vi "PM9_TCP_OPEN-SESSION.vi"(0 "VISA":refnum<visa-resource-name>="TCPIP0::169.254.70.190::502::SOCKET", 11 "error in (no error)":errorcluster) -> (6 "connection ID out":refnum<k5>, 15 "error out":errorcluster)   [LabVIEW 2018]
panel:
  in  "timeout ms ()":i32=5000
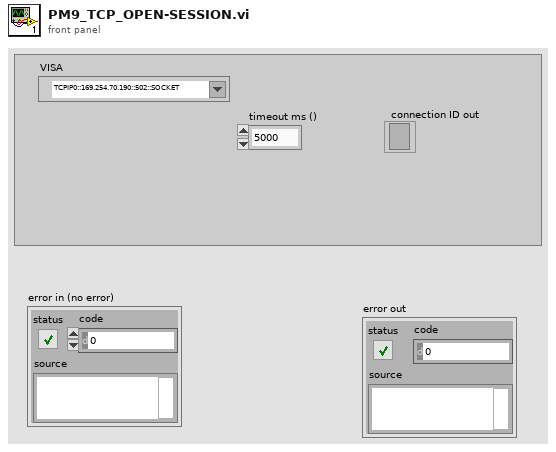
[diagram p1: front panel]
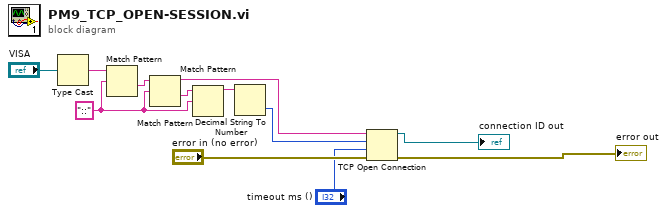
[diagram p0: block diagram]
diagram:
  w7 = "::" ("search string/char (-)")
  n1 = Type Cast(x="VISA") -> (*(type *) &x=w11:string)  [unwired: 1 in]
  n2 = Match Pattern(string=w11, regular expression=w7) -> (after substring=w10:string)  [unwired: 1 in, 3 out]
  n3 = Match Pattern(string=w10, regular expression=w7) -> (before substring=w9:string, after substring=w8:string)  [unwired: 1 in, 2 out]
  n4 = Match Pattern(string=w8, regular expression=w7) -> (before substring=w6:string)  [unwired: 1 in, 3 out]
  n5 = Decimal String To Number(string=w6) -> (number=w5:i32)  [unwired: 2 in, 1 out]
  n6 = TCP Open Connection(address=w9, remote port or service name=w5, timeout ms (60000)="timeout ms ()", error in (no error)="error in (no error)") -> (connection ID=→"connection ID out":refnum<k5>, error out=→"error out":errorcluster)  [unwired: 1 in]
